vi "Get Duplicated GU Number.vi"(8 "error in":errorcluster, 11 "GU Numbers":i32[](array[numeric])) -> (0 "error out":errorcluster, 2 "Repeated GU":cluster{"GU Number":i32, "Index":i32[]}[](array[cluster]))   [LabVIEW 2020, in "GUCalibration2.lvlib"]
uses:
  GUCalibration2.lvlib
  <vilib>/Utility/miscctls.llb/LVMapReplaceAction.ctl
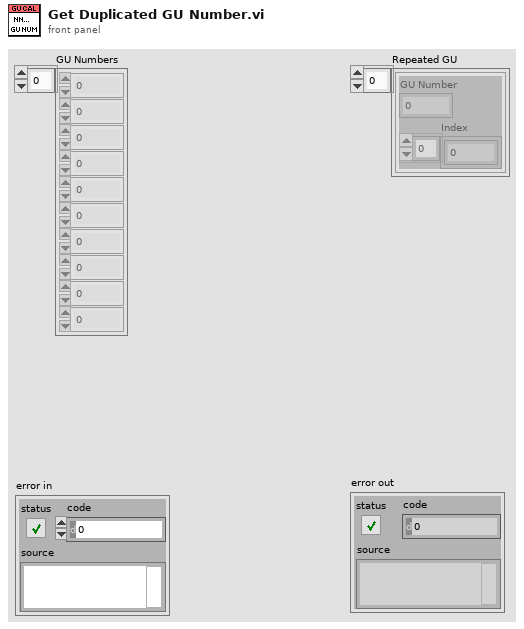
[diagram p1: front panel]
types:
  T1 = typedef "LVMapReplaceAction.ctl" = enum32{"Modify Entry only if found", "Add or Modify Entry", "Delete Entry"}
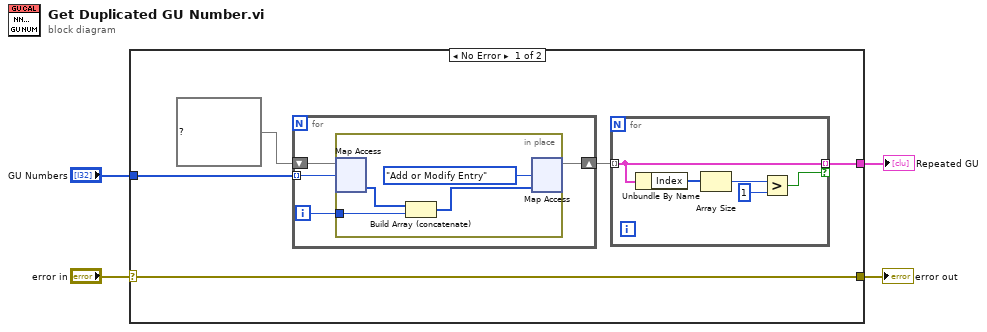
[diagram p0: block diagram]
diagram:
  n1 = case shown="No Error" "error in" {
    selector: "error in" -> [w6 w23]
    tunnel: "GU Numbers" -> [w8 _]
    tunnel: [w7 _] -> w3
    tunnel: [w6 w23] -> w1
    frame No Error {
      n2 = for {
        shift-right: [w16] -> w5
        shift-left: map{i32, i32[]} {} ("map") -> [w18]
        tunnel: w8 -> [w15] mode=indexing
        i -> [w17]
        n3 = in-place {
          in-place-border: w17 -> [w21]
          n4 = in-place-map #1(w18, w15) -> (w22:i32[])  [unwired: 1 in, 1 out]
          n5 = Build Array (concatenate)(w22, w21) -> (w20:i32[])
          n6 = in-place-map #1(w20, LVMapReplaceAction."Add or Modify Entry" ("action")) -> (w16:map{i32, i32[]})  [unwired: 2 out]
        }
      }
      n7 = for {
        tunnel: w5 -> [w11] mode=indexing
        tunnel: [w11] -> w7 mode=indexing if=w10
        n8 = Unbundle By Name(w11) -> ("Index"=w14:i32[])
        n9 = Array Size(array=w14) -> (size(s)=w13:i32)
        n10 = Greater?(x=w13, y=1) -> (0:w10:bool)
      }
    }
    frame Error {
    }
  }
  "error out" <- w1
  "Repeated GU" <- w3
